vi "filter_vec_bessel.vi"(5 "Order":i32=2, 6 "Fs":dbl, 7 "Reset":bool, 9 "LP cutoff":dbl=0.2 format="%0.3f", 10 "Initial value":dbl[](array[numeric]) format="%#_4g", 11 "Input X":dbl[](array[numeric]) format="%#_4g") -> (3 "Filtered X":dbl[](array[numeric]) format="%#_4g")   [LabVIEW 2012]
uses:
  <vilib>/Analysis/NI_AALBase.lvlib
panel:
  # "Will reset automatically if filter parameters change."
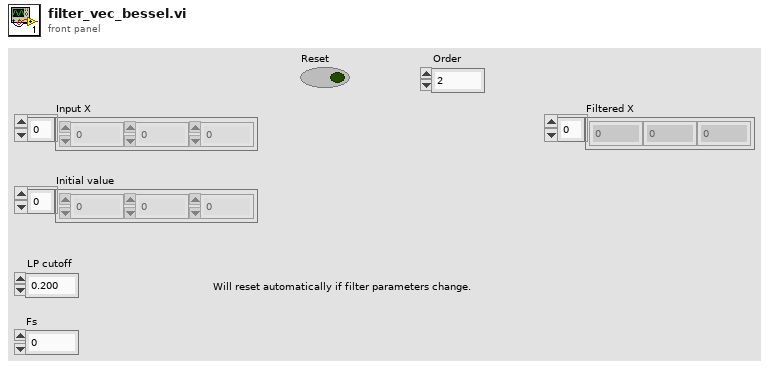
[diagram p1: front panel]
types:
  T1 = cluster{"filter structure":enum32{"IIR 2nd Order", "IIR 4th Order"}, "Reverse Coefficients":dbl[], "Forward Coefficients":dbl[]}
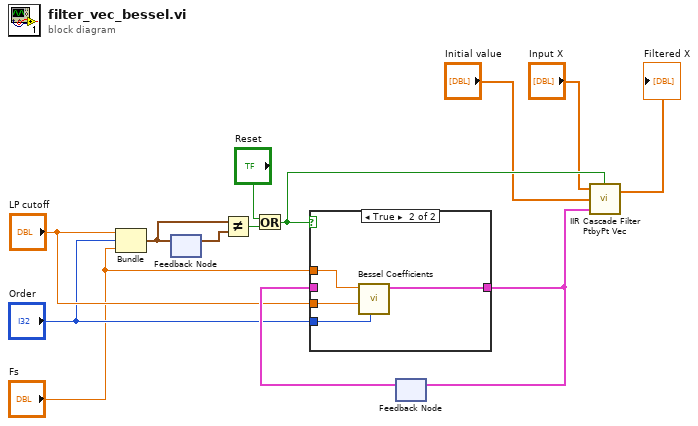
[diagram p0: block diagram]
diagram:
  n1 = Bundle("LP cutoff"="LP cutoff", "Order"="Order", "Fs"="Fs") -> (w8:cluster{"LP cutoff":dbl, "Order":i32, "Fs":dbl})  [unwired: 1 in]
  n2 = feedback #1() -> (w10:cluster{"LP cutoff":dbl, "Order":i32, "Fs":dbl})  [unwired: 1 in]
  n3 = feedback-in #1(w8) -> ()
  n4 = Not Equal?(x=w8, y=w10) -> (x != y?=w9:bool)
  n5 = Or(x="Reset", y=w9) -> (x .or. y?=w5:bool)
  n6 = feedback #2() -> (w13:T1)  [unwired: 1 in]
  n7 = case shown="True" w5 {
    tunnel: [w14 w18] -> w2
    tunnel: w13 -> [w14 _]
    tunnel: "LP cutoff" -> [_ w17]
    tunnel: "Order" -> [_ w16]
    tunnel: "Fs" -> [_ w15]
    frame False {
    }
    frame True {
      n8 = call <vilib>:"Bessel Coefficients.vi"("order"=w16, "low cutoff freq: fl"=w17, "sampling freq: fs"=w15) -> ("IIR Filter Cluster"=w18:T1)  [unwired: 7 in, 1 out]
    }
  }
  n9 = feedback-in #2(w2) -> ()
  n10 = call "IIR Cascade Filter PtbyPt Vec.vi"("initialize"=w5, "IIR Filter Cluster"=w2, "Initial value"="Initial value", "X"="Input X") -> ("Filtered X"=→"Filtered X":dbl[])  [unwired: 1 in]
